vi "UDP Data Link - Dialogs - Import Channel Paths Invalid.vi"(8 "error in (no error)":errorcluster, 11 "Item Names":string[](array[string])) -> (0 "error out":errorcluster)   [LabVIEW 2015, in "UDP Data Link System Explorer.lvlib"]
uses:
  UDP Data Link System Explorer.lvlib
panel:
  in  "Boolean":bool
  in  "Listbox":i32(listbox)
  # "The following channels were not able to be added because they \ndo not exist in the present system definition file:"
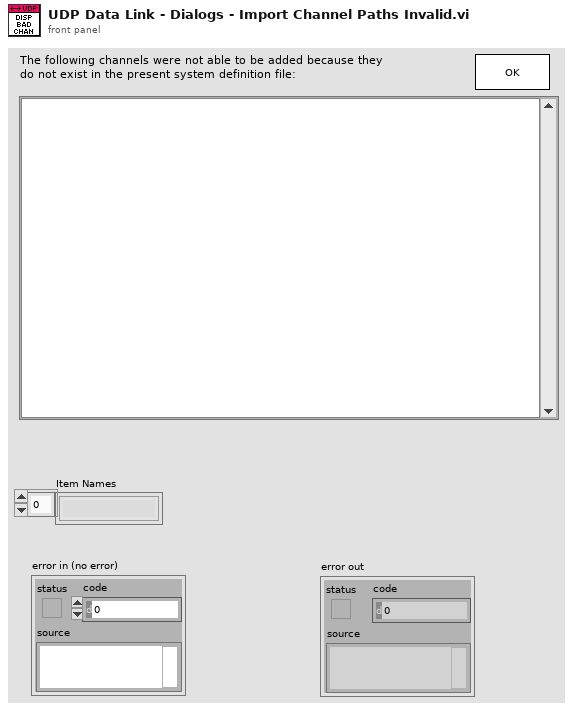
[diagram p1: front panel]
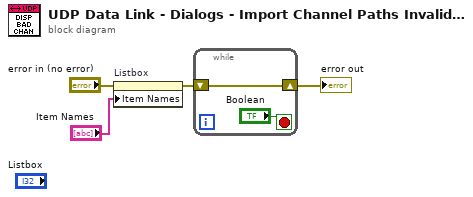
[diagram p0: block diagram]
diagram:
  n1 = property on="Listbox" class="LstBox (strict)"(error in="error in (no error)", "Item Names"="Item Names") -> (error out=w2:errorcluster)  [unwired: 1 in, 1 out]
  n2 = while {
    shift-right: [w5] -> w1
    shift-left: w2 -> [w5]
    stop <- "Boolean" stop-if-true
  }
  "error out" <- w1
